vi "populate_channel_tree.vi"(8 "error in (no error)":errorcluster, 9 "AI or AO":string, 10 "wiring config":string[][](array[string]), 11 "reference":refnum<vi>) -> (0 "error out":errorcluster, 3 "reference out":refnum<vi>)   [LabVIEW 2016]
uses:
  <vilib>/JDP Science/JDP Science Common Utilities/JDP Utility.lvlib
panel:
  out "subarray":string[](array[string])
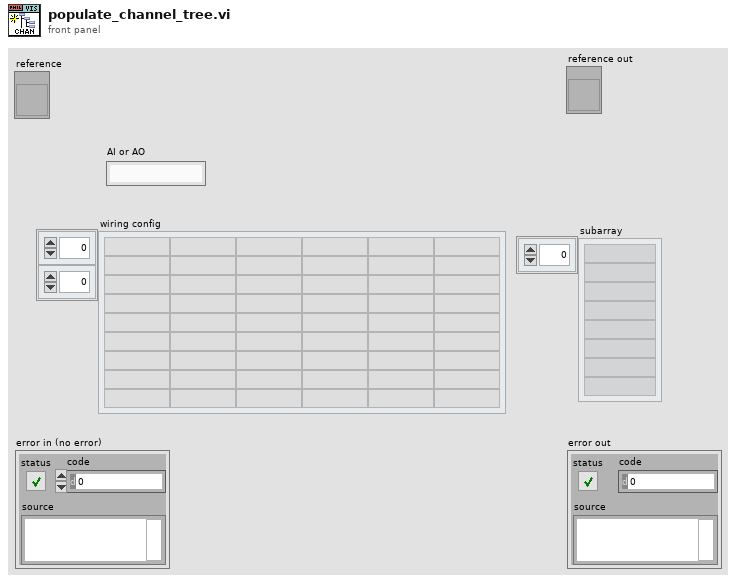
[diagram p1: front panel]
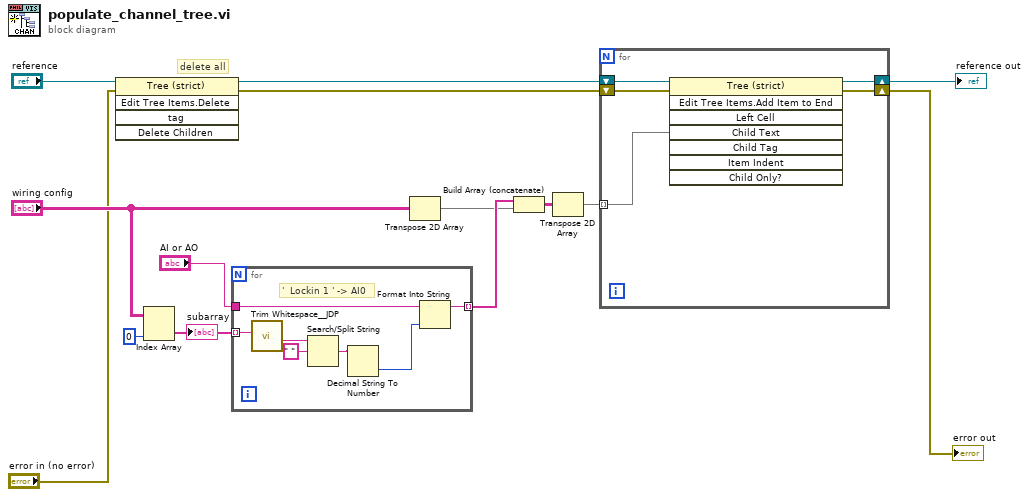
[diagram p0: block diagram]
diagram:
  # "delete all"
  n1 = invoke class="Tree (strict)" method="Edit Tree Items.Delete"(reference="reference", error in="error in (no error)") -> (reference out=w12:refnum<vi>, error out=w11:errorcluster)  [unwired: 3 in, 3 out]
  n2 = Index Array(array="wiring config", index (col)=0 ("disabled index (col)")) -> (element=w9:string[])  [unwired: 1 in]
  "subarray" <- w9
  n3 = for {
    tunnel: w9 -> [w21] mode=indexing
    tunnel: "AI or AO" -> [w15]
    tunnel: [w17] -> w5 mode=indexing
    # "'  Lockin 1 ' -> AI0"
    n4 = call <vilib>:"Trim Whitespace__JDP.vi"("String in"=w21) -> ("String out"=w18:string)  [unwired: 6 in]
    n5 = Search/Split String(string=w18, search string/char (-)=" ") -> (match + rest of string=w19:string)  [unwired: 1 in, 2 out]
    n6 = Decimal String To Number(string=w19) -> (number=w16:i32)  [unwired: 2 in, 1 out]
    n7 = Format Into String(initial string=w15, w16) -> (resulting string=w17:string)  [unwired: 2 in, 1 out]
  }
  n8 = Transpose 2D Array(2D array="wiring config") -> (transposed array=w3:string[][])
  n9 = Build Array (concatenate)(w5, w3) -> (w6:string[][])
  n10 = Transpose 2D Array(2D array=w6) -> (transposed array=w7:string[][])
  n11 = for {
    shift-right: [w26] -> w14
    shift-left: w12 -> [w25]
    tunnel: w7 -> [w23] mode=indexing
    shift-right: [w22] -> w1
    shift-left: w11 -> [w24]
    n12 = invoke on="Invoke Node" class="Tree (strict)" method="Edit Tree Items.Add Item to End"(reference=w25, error in=w24, "Child Text"=w23) -> (reference out=w26:refnum<vi>, error out=w22:errorcluster)  [unwired: 5 in, 6 out]
  }
  "reference out" <- w14
  "error out" <- w1
